vi "Read preset modes.vi"(8 "error in (no error)":errorcluster, 11 "S4GEI in":refnum<class "S4GEI.lvclass">) -> (0 "error out":errorcluster, 2 "preset modes":T1, 3 "S4GEI out":refnum<class "S4GEI.lvclass">)   [LabVIEW 2018, in "S4GEI.lvclass"]
uses:
  S4GEI.lvclass
  S4GEI.lvclass/S4GEI.ctl
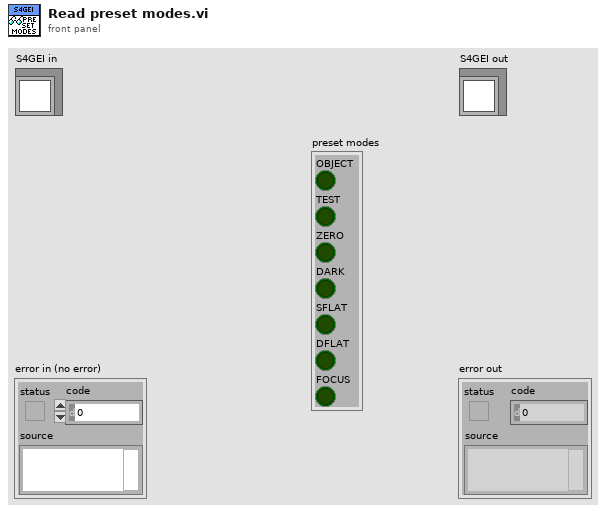
[diagram p1: front panel]
types:
  T1 = cluster{"OBJECT":bool, "TEST":bool, "ZERO":bool, "DARK":bool, "SFLAT":bool, "DFLAT":bool, "FOCUS":bool}
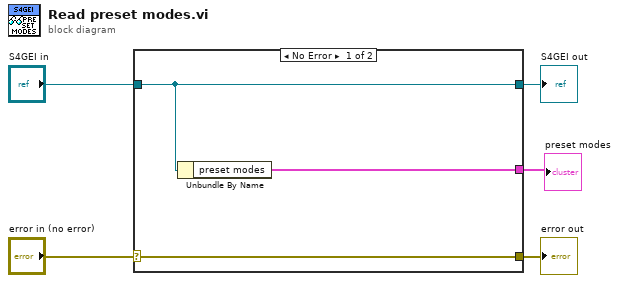
[diagram p0: block diagram]
diagram:
  n1 = case shown="No Error" "error in (no error)" {
    selector: "error in (no error)" -> [w8 w9]
    tunnel: [w8 w9] -> w4
    tunnel: [w7 w10] -> w2
    tunnel: "S4GEI in" -> [w7 w10]
    tunnel: [w6 _] -> w1
    frame No Error {
      n2 = Unbundle By Name(w7) -> ("preset modes"=w6:T1)
    }
    frame Error {
    }
  }
  "error out" <- w4
  "S4GEI out" <- w2
  "preset modes" <- w1
